vi "Ex2CamerasSame.vi"() -> ()   [LabVIEW 2010]
panel:
  in  "camera 2 name":string
  in  "camera 1 name":string
  in  "Store 2":bool
  in  "stop 2":bool
  in  "Store":bool
  in  "stop":bool
  in  "Exposure Camera 2":dbl=0.5 format="%.2f"
  in  "Exposure Camera 1":dbl=0.5 format="%.2f"
  out "error out":errorcluster
  in  "error in (no error)":errorcluster
  # "Ex2Cameras:\nThis example runs two cameras in focus mode.\nRemember to setup two cameras in the pvcam.ini\nfile."
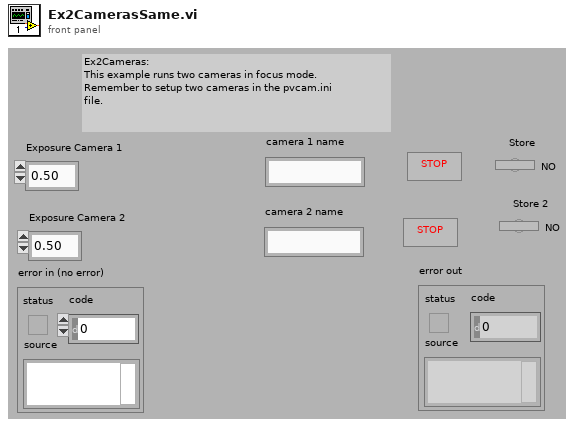
[diagram p1: front panel]
types:
  T1 = cluster{"Camera Handle":u32, "Pulser Handle":u32, "File Handle":u32, "Display Handle":u32, "Image Handle":u32}
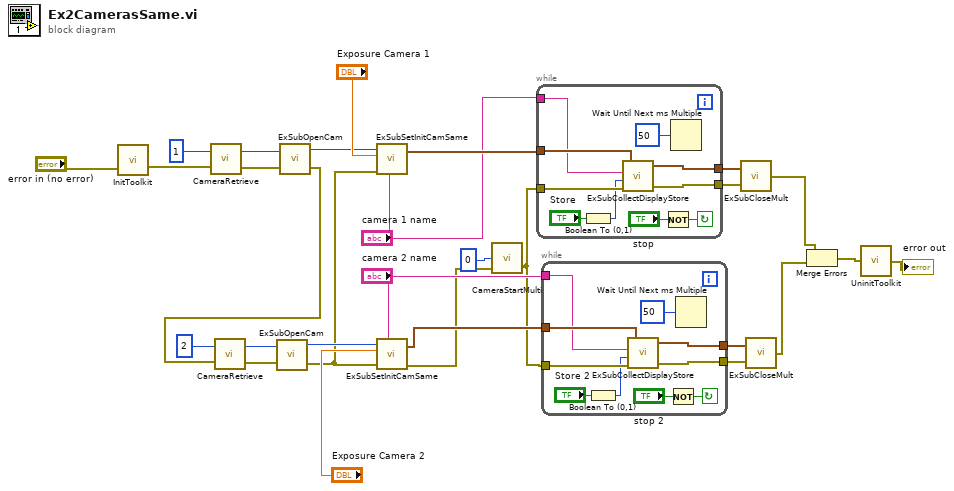
[diagram p0: block diagram]
diagram:
  n1 = call <userlib>:"InitToolkit.vi"("error in"="error in (no error)") -> ("error out"=w9:errorcluster)
  n2 = call <userlib>:"CameraRetrieve.vi"("error in"=w9, "Camera Index"=1) -> ("error out"=w11:errorcluster, "Device ID"=w10:u32)
  n3 = call "ExSubOpenCam.vi"("error in (no error)"=w11, "Camera Device ID"=w10) -> ("error out"=w5:errorcluster, "Camera Handle"=w18:u32)
  n4 = call <userlib>:"CameraRetrieve.vi"("error in"=w5, "Camera Index"=2) -> ("error out"=w6:errorcluster, "Device ID"=w7:u32)
  n5 = call "ExSubOpenCam.vi"("error in (no error)"=w6, "Camera Device ID"=w7) -> ("error out"=w12:errorcluster, "Camera Handle"=w17:u32)
  n6 = call "ExSubSetInitCamSame.vi"("Camera Handle"=w18, "Exposure"="Exposure Camera 1", "error in (no error)"=w12, "Name"="camera 1 name") -> ("Handles Out"=w21:T1)  [unwired: 1 in, 1 out]
  n7 = call "ExSubSetInitCamSame.vi"("Camera Handle"=w17, "Exposure"="Exposure Camera 2", "error in (no error)"=w12, "Name"="camera 2 name") -> ("Handles Out"=w22:T1, "error out"=w2:errorcluster)  [unwired: 1 in]
  n8 = call "CameraStartMulti.vi"("error in (no error)"=w2, "Number Of Cameras"=0) -> ("error out"=w1:errorcluster)  [unwired: 1 in, 1 out]
  n9 = while {
    tunnel: w21 -> [w38]
    tunnel: w1 -> [w37]
    tunnel: "camera 1 name" -> [w30]
    tunnel: [w35] -> w25
    tunnel: [w36] -> w26
    stop <- w33 continue-if-true
    n10 = Boolean To (0,1)(Boolean="Store") -> (0, 1=w31:i16)
    n11 = call "ExSubCollectDisplayStore.vi"("error in (no error)"=w37, "Store flag"=w31, "Display Title"=w30, "Handle Cluster"=w38) -> ("error out"=w35:errorcluster, "Handle Cluster Out"=w36:T1)  [unwired: 1 out]
    n12 = Not(x="stop") -> (.not. x?=w33:bool)
    n13 = Wait Until Next ms Multiple(millisecond multiple=u32 50) -> ()  [unwired: 1 out]
  }
  n14 = while {
    tunnel: w22 -> [w48]
    tunnel: w1 -> [w47]
    tunnel: "camera 2 name" -> [w40]
    tunnel: [w45] -> w23
    tunnel: [w46] -> w24
    stop <- w43 continue-if-true
    n15 = Boolean To (0,1)(Boolean="Store 2") -> (0, 1=w41:i16)
    n16 = call "ExSubCollectDisplayStore.vi"("error in (no error)"=w47, "Store flag"=w41, "Display Title"=w40, "Handle Cluster"=w48) -> ("error out"=w45:errorcluster, "Handle Cluster Out"=w46:T1)  [unwired: 1 out]
    n17 = Not(x="stop 2") -> (.not. x?=w43:bool)
    n18 = Wait Until Next ms Multiple(millisecond multiple=u32 50) -> ()  [unwired: 1 out]
  }
  n19 = call "ExSubCloseMult.vi"("error in (no error)"=w25, "Handles In"=w26) -> ("error out"=w14:errorcluster)
  n20 = call "ExSubCloseMult.vi"("error in (no error)"=w23, "Handles In"=w24) -> ("error out"=w13:errorcluster)
  n21 = Merge Errors(w14, w13) -> (w16:errorcluster)
  n22 = call <userlib>:"UninitToolkit.vi"("error in"=w16) -> ("error out"=→"error out":errorcluster)
